vi "IMAQdx Switch Camera Driver.vi"(8 "error in":errorcluster, 10 "Driver Description":string="NI-IMAQdx IIDC Digital Camera", 11 "Driver Name":string="{6BDD1FC6-810F-11D0-BEC7-08002BE2092F}") -> (0 "error out":errorcluster)   [LabVIEW 2020, in "NI_Vision_Acquisition_Software.lvlib"]
doc: "Switch driver for specified camera."
uses:
  NI_Vision_Acquisition_Software.lvlib
  niimaqdx.dll
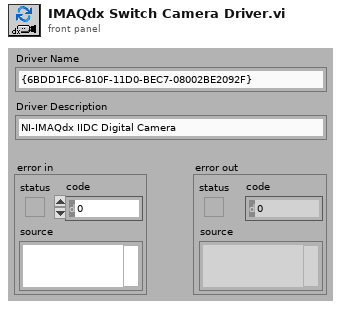
[diagram p1: front panel]
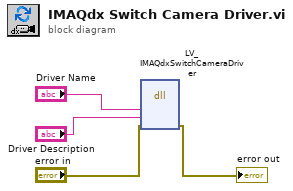
[diagram p0: block diagram]
diagram:
  n1 = dll-call lib="niimaqdx.dll" fn="LV_IMAQdxSwitchCameraDriver"("driverName"="Driver Name", "driverDescription"="Driver Description", "error in"="error in") -> ("error in"=→"error out":errorcluster)  [unwired: 6 in, 2 out]
